vi "Hierarchy Example VI.vi"   [LabVIEW 2026]
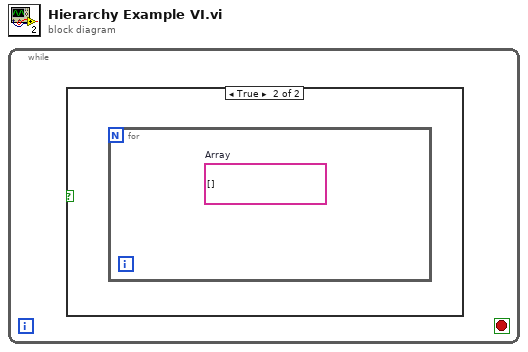
[diagram p0: block diagram]
diagram:
  n1 = while {
    stop <- _ stop-if-true
    n2 = case shown="True" {
      selector: _ -> [_ _]
      frame False {
      }
      frame True {
        n3 = for {
          (unwired) string[] []  # Array
        }
      }
    }
  }
